vi "Null Broadcast Events--constant.vi"() -> (3 "Monedas Broadcast Events":T1)   [LabVIEW 2019, in "Monedas.lvlib"]
doc: "Returns the broadcast events cluster with null references for defining the event types in a Register For Events function.\n_____\nBased on DQMH Project Template 6.1.0.94."
uses:
  Monedas.lvlib
  Users/pcort/Documents/github/dqmh-exercise-03/Libraries/My Singleton Module/Broadcast Events--cluster.ctl
  Users/pcort/Documents/github/dqmh-exercise-03/Libraries/My Singleton Module/Did Init Argument--cluster.ctl
  Users/pcort/Documents/github/dqmh-exercise-03/Libraries/My Singleton Module/Status Updated Argument--cluster.ctl
  Users/pcort/Documents/github/dqmh-exercise-03/Libraries/My Singleton Module/Error Reported Argument--cluster.ctl
  Users/pcort/Documents/github/dqmh-exercise-03/Libraries/My Singleton Module/Do Something Argument--cluster.ctl
  Users/pcort/Documents/github/dqmh-exercise-03/Libraries/My Singleton Module/Stop Argument--cluster.ctl
  Users/pcort/Documents/github/dqmh-exercise-03/Libraries/My Singleton Module/Get Module Execution Status Argument--cluster.ctl
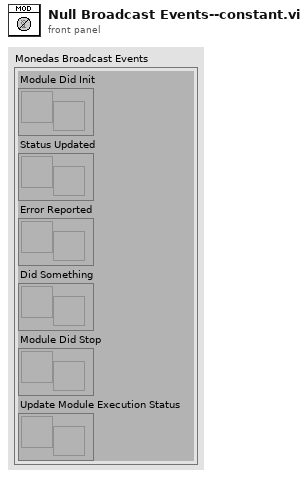
[diagram p1: front panel]
types:
  T1 = typedef "Monedas.lvlib/Broadcast Events--cluster.ctl" = cluster{"Module Did Init":refnum<user-event>, "Status Updated":refnum<user-event>, "Error Reported":refnum<user-event>, "Did Something":refnum<user-event>, "Module Did Stop":refnum<user-event>, "Update Module Execution Status":refnum<user-event>}
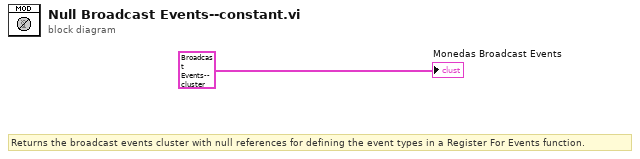
[diagram p0: block diagram]
diagram:
  # "Returns the broadcast events cluster with null references for defining the event types in a Register For Events function."
  "Monedas Broadcast Events" <- T1 {"Module Did Init"=refnum, "Status Updated"=refnum, "Error Reported"=refnum, "Did Something"=refnum, "Module Did Stop"=refnum, "Update Module Execution Status"=refnum} ("Broadcast Events")
